vi "Is Single Cluster in Ctrl Refs Array.vi"(11 "Refnums":refnum<vi>[](array[refnum])) -> (2 "error out":errorcluster, 3 "is error cluster?":bool)   [LabVIEW 2020]
uses:
  <vilib>/addons/analyzer/_analyzerutils.llb/VIAnUtil Check Type If ErrClust.vi
  <vilib>/Utility/Data Type/NI_Data Type.lvlib
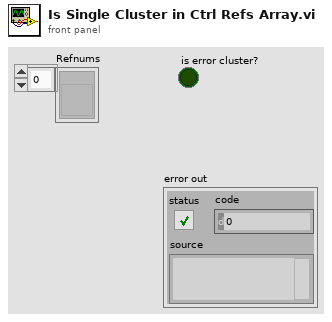
[diagram p1: front panel]
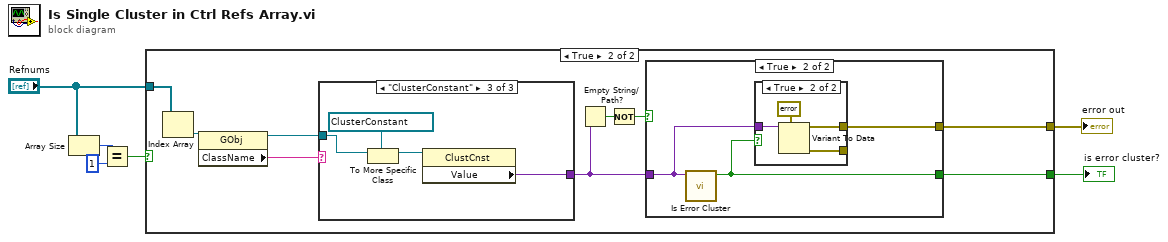
[diagram p0: block diagram]
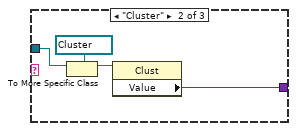
[diagram p6: hidden frame]
diagram:
  n1 = Array Size(array="Refnums") -> (size(s)=w1:i32)
  n2 = Equal?(x=w1, y=1) -> (x = y?=w3:bool)
  n3 = case shown="True" w3 {
    tunnel: "Refnums" -> [_ w14]
    tunnel: [_ w11] -> w5
    tunnel: [_ w10] -> w6
    frame False {
    }
    frame True {
      n4 = Index Array(array=w14) -> (element=w15:refnum<vi>)  [unwired: 1 in]
      n5 = property class="GObj"(reference=w15) -> (reference out=w13:refnum<vi>, "ClassName"=w12:string)  [unwired: 1 in, 1 out]
      n6 = case shown="\"ClusterConstant\"" w12 {
        tunnel: w13 -> [_ w25 w29]
        tunnel: [_ w23 w27] -> w9
        frame Default {
        }
        frame "Cluster" {
          n7 = To More Specific Class(target class=refnum<vi> refnum ("reference out"), reference=w25) -> (specific class reference=w24:refnum<vi>)  [unwired: 1 in, 1 out]
          n8 = property class="Clust"(reference=w24) -> ("Value"=w23:variant)  [unwired: 1 in, 2 out]
        }
        frame "ClusterConstant" {
          n9 = To More Specific Class(target class=refnum<vi> refnum ("reference out"), reference=w29) -> (specific class reference=w28:refnum<vi>)  [unwired: 1 in, 1 out]
          n10 = property class="ClustCnst"(reference=w28) -> ("Value"=w27:variant)  [unwired: 1 in, 2 out]
        }
      }
      n11 = Empty String/Path?(string/path=w9) -> (empty?=w8:bool)
      n12 = Not(x=w8) -> (.not. x?=w7:bool)
      n13 = case shown="True" w7 {
        tunnel: [_ w18] -> w11
        tunnel: [_ w17] -> w10
        tunnel: w9 -> [_ w16]
        frame False {
        }
        frame True {
          n14 = call <vilib>:"Is Error Cluster.vi"("variant"=w16) -> ("is error cluster?"=w18:bool)  [unwired: 9 in, 1 out]
          n15 = case shown="True" w18 {
            tunnel: w16 -> [_ w21]
            tunnel: [_ w20] -> w17
            tunnel: [_ w19] -> _
            frame False {
            }
            frame True {
              n16 = Variant To Data(type=errorcluster {"status"=FALSE, "code"=0, "source"=""} ("error out"), Variant=w21) -> (data=w20:errorcluster, error out=w19:errorcluster)  [unwired: 1 in]
            }
          }
        }
      }
    }
  }
  "error out" <- w6
  "is error cluster?" <- w5
